vi "BotSpeak_RunWaitScript.vi"(2 "Subroutine (runs prgm if unwired)":string, 3 "Bot Settings":T1) -> (0 "response":string="169.254.32.85", 1 "Bot Settings":T1)   [LabVIEW 2012]
doc: "Runs scripted code that has been loaded onto the hardware with a Load VI."
uses:
  <userlib>/botspeak/VIs/Direct/BotSpeak_Control.ctl
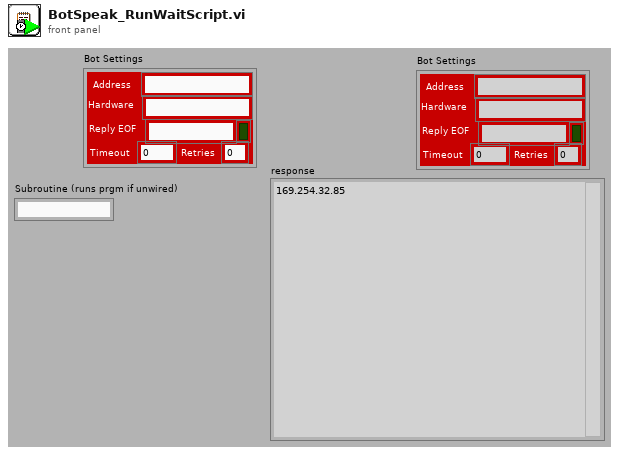
[diagram p1: front panel]
types:
  T1 = typedef "BotSpeak_Control.ctl" = cluster{"Address":string, "Reply EOF":string, "Hardware":string, "Retries":i8, "Timeout":i32, "Open?":bool}
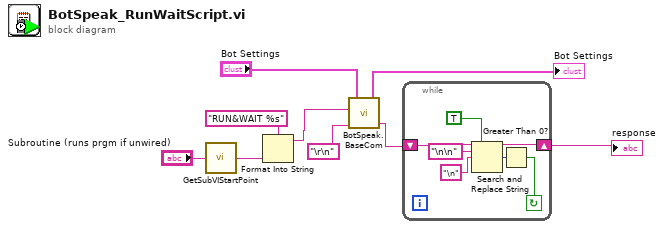
[diagram p0: block diagram]
diagram:
  n1 = call <userlib>:"GetSubVIStartPoint.vi"("Subroutine (runs prgm if unwired)"="Subroutine (runs prgm if unwired)") -> ("String"=w4:string)
  n2 = Format Into String(format string="RUN&WAIT %s" ("command"), w4) -> (resulting string=w3:string)  [unwired: 2 in, 1 out]
  n3 = call <userlib>:"BotSpeak.BaseCom.vi"("Termination"="\r\n", "command"=w3, "Bot Settings in"="Bot Settings") -> ("response"=w2:string, "Bot Settings out"=→"Bot Settings":T1)  [unwired: 2 in]
  n4 = while {
    shift-right: [w15] -> w1
    shift-left: w2 -> [w16]
    stop <- w10 continue-if-true
    n5 = Search and Replace String(replace all?=TRUE ("replace all? (F)"), input string=w16, search string="\n\n", replace string="\n" ("search string")) -> (result string=w15:string, number of replacements=w11:i32)  [unwired: 4 in, 2 out]
    n6 = Greater Than 0?(x=w11) -> (x > 0?=w10:bool)
  }
  "response" <- w1
